vi "关键参数区.vi"(11 "数组":u16[](array[numeric]) format="%04xH") -> (3 "关键参数区":T1)   [LabVIEW 2016, in "氨氮.lvlib"]
panel:
  # "共占用56 WORD"
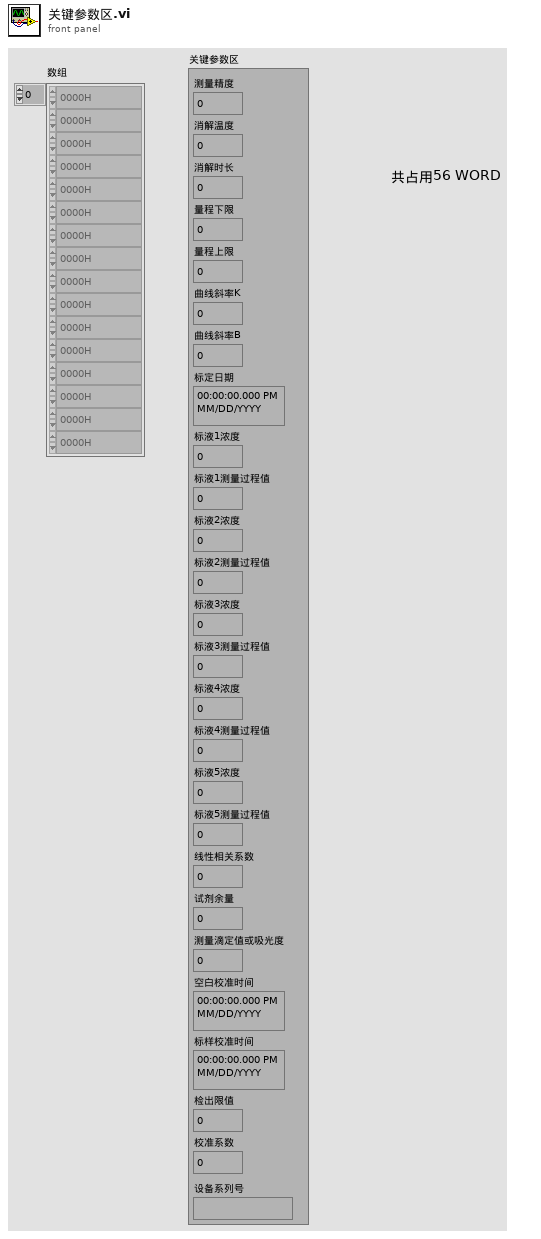
[diagram p1: front panel]
types:
  T1 = cluster{"测量精度":u16, "消解温度":u16, "消解时长":u16, "量程下限":sgl, "量程上限":sgl, "曲线斜率K":sgl, "曲线斜率B":sgl, "标定日期":timestamp, "标液1浓度":sgl, "标液1测量过程值":sgl, "标液2浓度":sgl, "标液2测量过程值":sgl, "标液3浓度":sgl, "标液3测量过程值":sgl, "标液4浓度":sgl, "标液4测量过程值":sgl, "标液5浓度":sgl, "标液5测量过程值":sgl, "线性相关系数":sgl, "试剂余量":u32, "测量滴定值或吸光度":sgl, "空白校准时间":timestamp, "标样校准时间":timestamp, "检出限值":sgl, "校准系数":sgl, "设备系列号":string}
  T2 = cluster{"WORD":u16, "WORD":u16, "WORD":u16, "FLOAT":sgl, "FLOAT":sgl, "FLOAT":sgl, "FLOAT":sgl, "time stamp":timestamp, "FLOAT":sgl, "FLOAT":sgl, "FLOAT":sgl, "FLOAT":sgl, "FLOAT":sgl, "FLOAT":sgl, "FLOAT":sgl, "FLOAT":sgl, "FLOAT":sgl, "FLOAT":sgl, "FLOAT":sgl, "DWORD":i32, "FLOAT":sgl, "time stamp":timestamp, "time stamp":timestamp, "FLOAT":sgl, "FLOAT":sgl, "string":string}
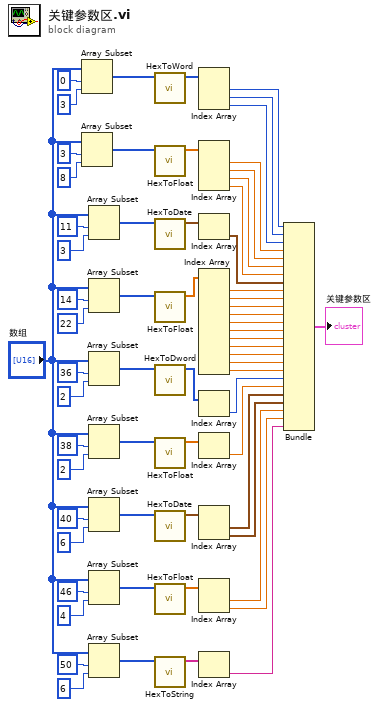
[diagram p0: block diagram]
diagram:
  n1 = Array Subset(array="数组", index=0 ("索引"), length=3 ("长度")) -> (w59:u16[])
  n2 = Array Subset(array="数组", index=3 ("索引"), length=8 ("长度")) -> (w55:u16[])
  n3 = Array Subset(array="数组", index=11 ("索引"), length=3 ("长度")) -> (w47:u16[])
  n4 = Array Subset(array="数组", index=14 ("索引"), length=22 ("长度")) -> (w42:u16[])
  n5 = Array Subset(array="数组", index=36 ("索引"), length=2 ("长度")) -> (w17:u16[])
  n6 = Array Subset(array="数组", index=38 ("索引"), length=2 ("长度")) -> (w18:u16[])
  n7 = Array Subset(array="数组", index=40 ("索引"), length=6 ("长度")) -> (w30:u16[])
  n8 = Array Subset(array="数组", index=46 ("索引"), length=4 ("长度")) -> (w25:u16[])
  n9 = Array Subset(array="数组", index=50 ("索引"), length=6 ("长度")) -> (w19:u16[])
  n10 = call "HexToWord.vi"("数组"=w59) -> ("WORD"=w58:u16[])  [unwired: 10 in]
  n11 = call "HexToFloat.vi"("数组"=w55) -> ("FLOAT"=w54:sgl[])  [unwired: 10 in]
  n12 = call "HexToDate.vi"("数组"=w47) -> ("DATE"=w46:timestamp[])  [unwired: 10 in]
  n13 = call "HexToFloat.vi"("数组"=w42) -> ("FLOAT"=w41:sgl[])  [unwired: 10 in]
  n14 = call "HexToDword.vi"("数组"=w17) -> ("DWORD"=w36:i32[])  [unwired: 10 in]
  n15 = call "HexToFloat.vi"("数组"=w18) -> ("FLOAT"=w13:sgl[])  [unwired: 10 in]
  n16 = call "HexToDate.vi"("数组"=w30) -> ("DATE"=w29:timestamp[])  [unwired: 10 in]
  n17 = call "HexToFloat.vi"("数组"=w25) -> ("FLOAT"=w23:sgl[])  [unwired: 10 in]
  n18 = call "HexToString.vi"("数组"=w19) -> ("STRING"=w2:string[])  [unwired: 10 in]
  n19 = Index Array(array=w58) -> (element #1=w62:u16, element #2=w61:u16, element #3=w60:u16)  [unwired: 3 in]
  n20 = Index Array(array=w54) -> (element #1=w53:sgl, element #2=w52:sgl, element #3=w51:sgl, element #4=w50:sgl)  [unwired: 4 in]
  n21 = Index Array(array=w46) -> (element=w45:timestamp)  [unwired: 1 in]
  n22 = Index Array(array=w41) -> (element #1=w40:sgl, element #2=w39:sgl, element #3=w38:sgl, element #4=w37:sgl, element #5=w10:sgl, element #6=w9:sgl, element #7=w8:sgl, element #8=w7:sgl, element #9=w6:sgl, element #10=w5:sgl, element #11=w4:sgl)  [unwired: 11 in]
  n23 = Index Array(array=w36) -> (element=w33:i32)  [unwired: 1 in]
  n24 = Index Array(array=w13) -> (element=w12:sgl)  [unwired: 1 in]
  n25 = Index Array(array=w29) -> (element #1=w28:timestamp, element #2=w27:timestamp)  [unwired: 2 in]
  n26 = Index Array(array=w23) -> (element #1=w22:sgl, element #2=w11:sgl)  [unwired: 2 in]
  n27 = Index Array(array=w2) -> (element=w1:string)  [unwired: 1 in]
  n28 = Bundle("WORD"=w62, "WORD"=w61, "WORD"=w60, "FLOAT"=w53, "FLOAT"=w52, "FLOAT"=w51, "FLOAT"=w50, "time stamp"=w45, "FLOAT"=w40, "FLOAT"=w39, "FLOAT"=w38, "FLOAT"=w37, "FLOAT"=w10, "FLOAT"=w9, "FLOAT"=w8, "FLOAT"=w7, "FLOAT"=w6, "FLOAT"=w5, "FLOAT"=w4, "DWORD"=w33, "FLOAT"=w12, "time stamp"=w28, "time stamp"=w27, "FLOAT"=w22, "FLOAT"=w11, "string"=w1) -> (→"关键参数区":T2)  [unwired: 1 in]
